vi "flip_array_vertical.vi"(11 "Array in":u8[][](array[numeric])) -> (3 "Array out":u8[][](array[numeric]))   [LabVIEW 2025]
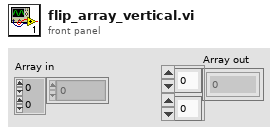
[diagram p1: front panel]
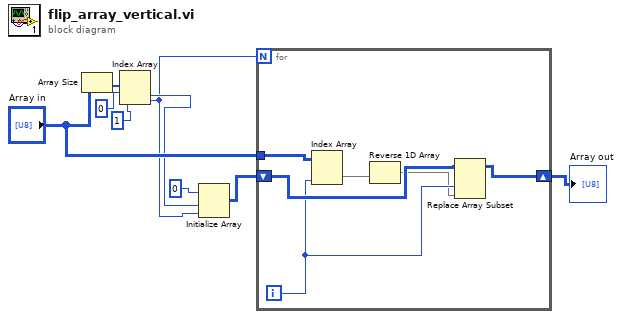
[diagram p0: block diagram]
diagram:
  n1 = Array Size(array="Array in") -> (size(s)=w9:i32[])
  n2 = Index Array(array=w9, index #1=0 ("index"), index #2=1 ("index")) -> (element #1=w2:i32, element #2=w1:i32)
  n3 = Initialize Array(u8 0 ("element"), w2, w1) -> (w7:u8[][])
  n4 = for {
    N: w1 -> [_]
    tunnel: "Array in" -> [w15]
    shift-right: [w13] -> w5
    shift-left: w7 -> [w12]
    i -> [w11]
    n5 = Index Array(array=w15, index (col)=w11) -> (element=w14:u8[])  [unwired: 1 in]
    n6 = Reverse 1D Array(array=w14) -> (reversed array=w10:u8[])
    n7 = Replace Array Subset(array=w12, new element=w10, index (col)=w11) -> (w13:u8[][])  [unwired: 1 in]
  }
  "Array out" <- w5
